vi "Benchmark.vi"() -> ()   [LabVIEW 2018, in "TwinCAT ADS.lvclass"]
uses:
  TwinCAT ADS.lvclass
panel:
  out "Value":variant
  out "Values":variant[](array[variant])
  in  "stop":bool
  out "Time(s)":dbl format="%^#_6e"
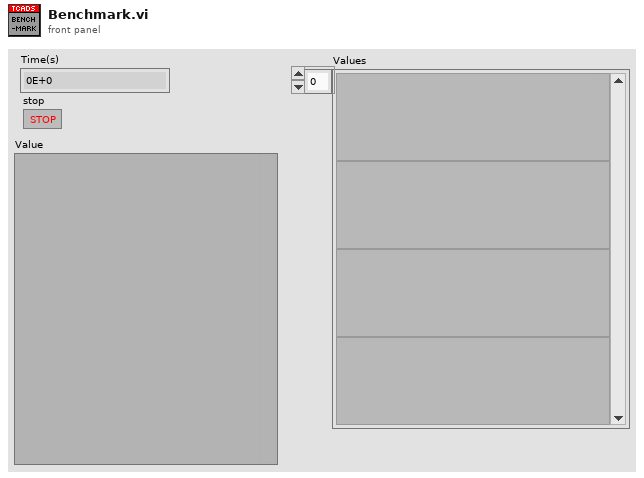
[diagram p1: front panel]
types:
  T1 = cluster{"_bMember":bool, "_nMember":i32, "_sMember":string}
  T2 = cluster{"status":bool, "time stamp":timestamp, dbl}
  T3 = cluster{string, bool, "time stamp":timestamp, dbl}
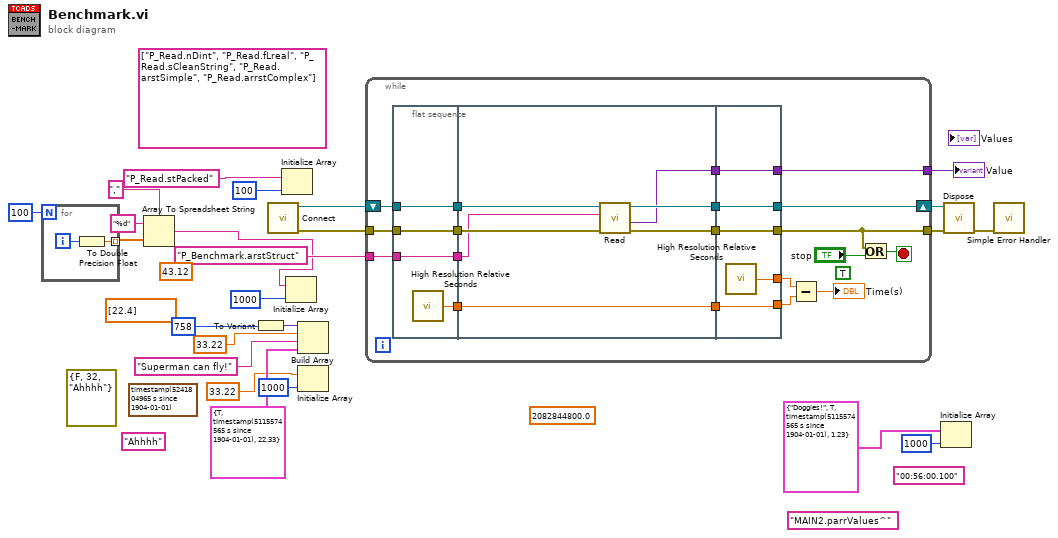
[diagram p0: block diagram]
diagram:
  (unwired) 2082844800.0 ("double precision float")
  (unwired) timestamp(5241804965 s since 1904-01-01) ("time stamp")
  (unwired) "Ahhhh" ("_sMember")
  (unwired) T1 {"_bMember"=FALSE, "_nMember"=32, "_sMember"="Ahhhh"} ("FB_Simple")
  (unwired) dbl[] [22.4]
  (unwired) 43.12
  (unwired) string[] ["P_Read.nDint", "P_Read.fLreal", "P_Read.sCleanString", "P_Read.arstSimple", "P_Read.arrstComplex"]
  (unwired) "00:56:00.100"
  (unwired) "MAIN2.parrValues^"
  n1 = for {
    N: 100 -> [_]
    tunnel: [w25] -> w8 mode=indexing
    i -> [w26]
    n2 = To Double Precision Float(number=w26) -> (double precision float=w25:dbl)
  }
  n3 = Array To Spreadsheet String(delimiter (Tab)=",", array=w8, 3:"%d" ("format string")) -> (spreadsheet string=w5:string)
  n4 = To Variant(anything=758) -> (Variant=w17:variant)
  n5 = call "Connect.vi"() -> ("error out"=w21:errorcluster, "TwinCAT ADS out"=w22:refnum<class "TwinCAT ADS.lvclass">)  [unwired: 10 in]
  n6 = Initialize Array("P_Read.stPacked", 100 ("dimension size")) -> ()  [unwired: 1 out]
  n7 = Initialize Array(w5, 1000 ("dimension size")) -> ()  [unwired: 1 out]
  n8 = Build Array(w17, 33.22, "Superman can fly!", T2 {"status"=TRUE, "time stamp"=timestamp(5115574565 s since 1904-01-01), 22.33} ("error constant")) -> ()  [unwired: 1 out]
  n9 = Initialize Array(33.22, 1000 ("dimension size")) -> ()  [unwired: 1 out]
  n10 = while {
    shift-right: [w34] -> w23
    shift-left: w22 -> [w41]
    tunnel: w21 -> [w40]
    tunnel: [w32] -> w24
    tunnel: "P_Benchmark.arstStruct" -> [w30]
    tunnel: [w28] -> w1
    stop <- w33 stop-if-true
    (unwired) TRUE
    n11 = flat-sequence {
      tunnel: w41 -> [w48]
      tunnel: w40 -> [w49]
      tunnel: [w49] -> w45
      tunnel: [w48] -> w44
      tunnel: [w47] -> w43
      tunnel: [w46] -> w31
      tunnel: w30 -> [w46]
      tunnel: w45 -> [w52]
      tunnel: w44 -> [w55]
      tunnel: w43 -> [w56]
      tunnel: [w56] -> w42
      tunnel: [w54] -> w36
      tunnel: [w53] -> w35
      tunnel: w31 -> [w51]
      tunnel: [w50] -> w29
      tunnel: w42 -> [w61]
      tunnel: [w61] -> w38
      tunnel: [w60] -> w39
      tunnel: w36 -> [w59]
      tunnel: w35 -> [w58]
      tunnel: [w59] -> w34
      tunnel: [w58] -> w32
      tunnel: w29 -> [w57]
      tunnel: [w57] -> w28
      frame #0 {
        n12 = call <vilib>:"High Resolution Relative Seconds.vi"() -> ("relative seconds"=w47:dbl)
      }
      frame #1 {
        n13 = call "Read.vi"("error in (no error)"=w52, "Symbol Name"=w51, "TwinCAT ADS in"=w55) -> ("error out"=w53:errorcluster, "Value"=w50:variant, "TwinCAT ADS out"=w54:refnum<class "TwinCAT ADS.lvclass">)  [unwired: 6 in]
      }
      frame #2 {
        n14 = call <vilib>:"High Resolution Relative Seconds.vi"() -> ("relative seconds"=w60:dbl)
      }
    }
    n15 = Subtract(x=w39, y=w38) -> (x-y=→"Time(s)":dbl)
    n16 = Or(x=w32, y="stop") -> (x .or. y?=w33:bool)
  }
  "Value" <- w1
  n17 = Initialize Array(T3 {"Doggies!", TRUE, "time stamp"=timestamp(5115574565 s since 1904-01-01), 1.23}, 1000 ("dimension size")) -> ()  [unwired: 1 out]
  n18 = call "Dispose.vi"("error in (no error)"=w24, "TwinCAT ADS in"=w23) -> ("error out"=w20:errorcluster)  [unwired: 9 in]
  n19 = call <vilib>:"Simple Error Handler.vi"("error in (no error)"=w20) -> ()  [unwired: 4 in, 5 out]
